vi "Update Cursor State.vi"(8 "error in (no error)":errorcluster, 10 "Cursor State":T1 {"Y" format="%#_6p"; "X" format="%#_6p"}, 11 "Cursor Digitizer in":refnum<class "Cursor Digitizer.lvclass">) -> (0 "error out":errorcluster, 3 "Cursor Digitizer out":refnum<class "Cursor Digitizer.lvclass">)   [LabVIEW 2019, in "Cursor Digitizer.lvclass"]
uses:
  Cursor Digitizer.lvclass
  Cursor State.ctl
  Cursor Digitizer.lvclass/Cursor Digitizer.ctl
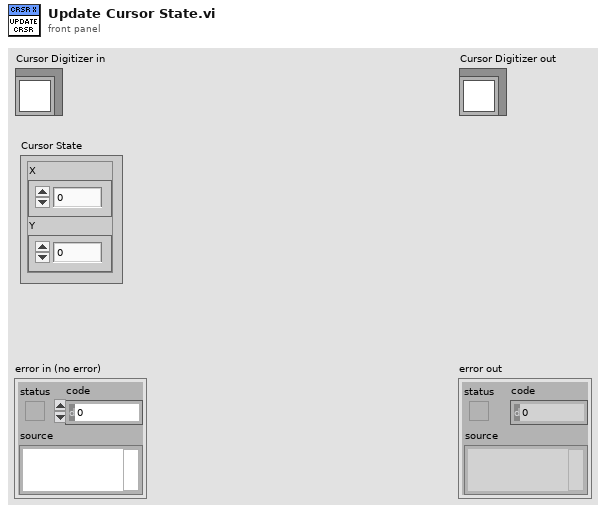
[diagram p1: front panel]
types:
  T1 = typedef "Cursor State.ctl" = cluster{"X":dbl, "Y":dbl}
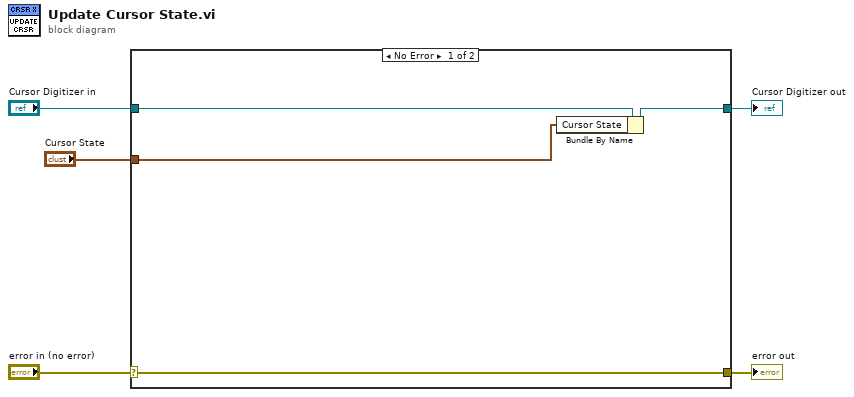
[diagram p0: block diagram]
diagram:
  n1 = case shown="No Error" "error in (no error)" {
    selector: "error in (no error)" -> [w8 w11]
    tunnel: [w8 w11] -> w4
    tunnel: [w7 w10] -> w2
    tunnel: "Cursor Digitizer in" -> [w9 w10]
    tunnel: "Cursor State" -> [w6 _]
    frame No Error {
      n2 = Bundle By Name(cluster=w9, "Cursor State"=w6) -> (w7:refnum<class "Cursor Digitizer.lvclass">)
    }
    frame Error {
    }
  }
  "error out" <- w4
  "Cursor Digitizer out" <- w2
